vi "NBFM Modulation Demo (Single Tone) - Basic.vi"() -> ()   [LabVIEW 2013]
uses:
  <vilib>/addons/Modulation/Analog/MT Passband PLL.vi
  <vilib>/express/express analysis/Spectral/Block/exnSpectralBlock spectral measurements power poly.vi
  <vilib>/express/express analysis/Spectral/Block/exnSpectralBlock spectral measurements power DDT.vi
  <vilib>/express/express analysis/Spectral/XNode/ExpressSpectralMeasurementsBlockNode.xnode
  <vilib>/addons/Modulation/niAMT.lvlib
panel:
  out "estimated carrier frequency (Hz)":dbl
  in  "Mod. Freq.":dbl=2000.0 caption="Frequency"
  in  "WAV SR":dbl=44100.0 caption="dt"
  in  "LPF Cut-Off":dbl=10000.0 caption="Lower Cut-Off"
  in  "AWGN (dB)":dbl(slide)=30.0 caption="Standard deviation" scale=-20.0..50.0
  out "Recovered Signal":dynamicdata(graph)
  out "Baseband":dynamicdata(graph)
  out "FM FFT":dynamicdata(graph)
  out "FM Wave":dynamicdata(graph)
  in  "Carrier Amp.":dbl=1.0 caption="Amplitude"
  in  "stop":bool
  in  "Frequency Deviation":dbl(slide)=400.0 scale=0.0..400.0
  in  "Carrier Freq.":dbl=100000.0 caption="Frequency"
  # "Frequency Modulation"
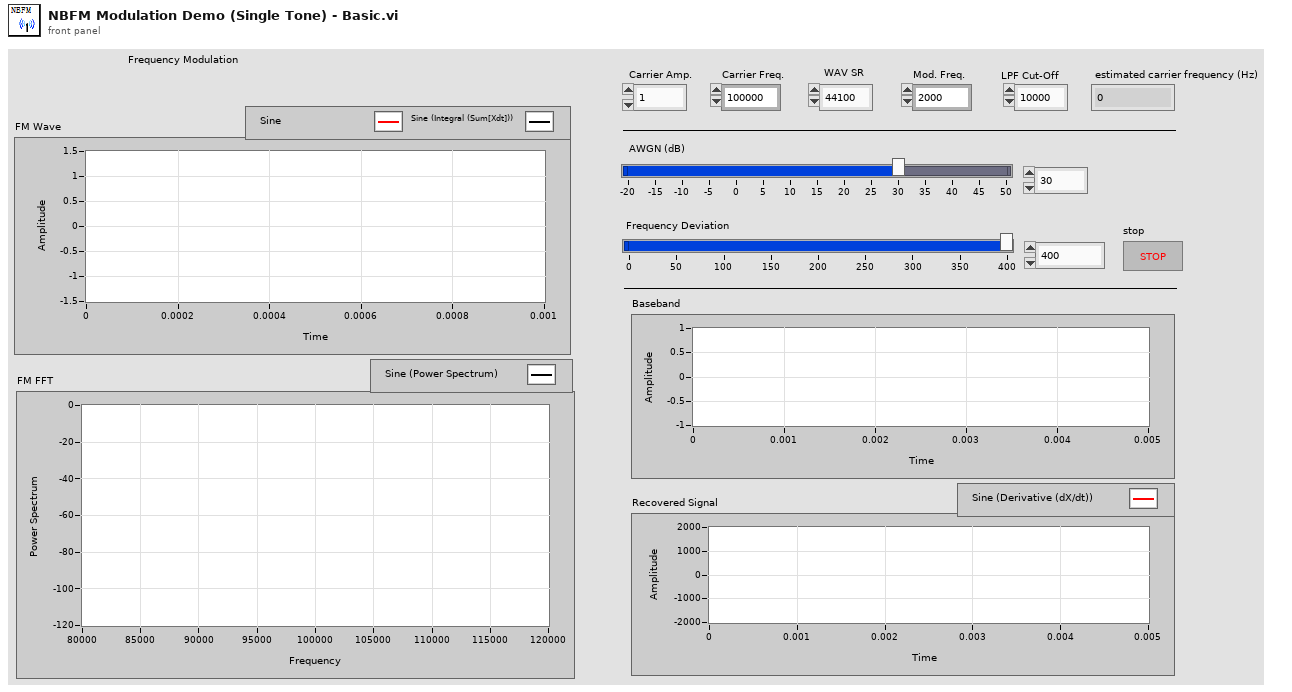
[diagram p1: front panel]
types:
  T1 = cluster{"averaging mode":u16, "weighting mode":u16, "number of averages":u32}
  T2 = cluster{"dB On (F)":bool, "unwrap phase (F)":bool, "convert to degree (F)":bool}
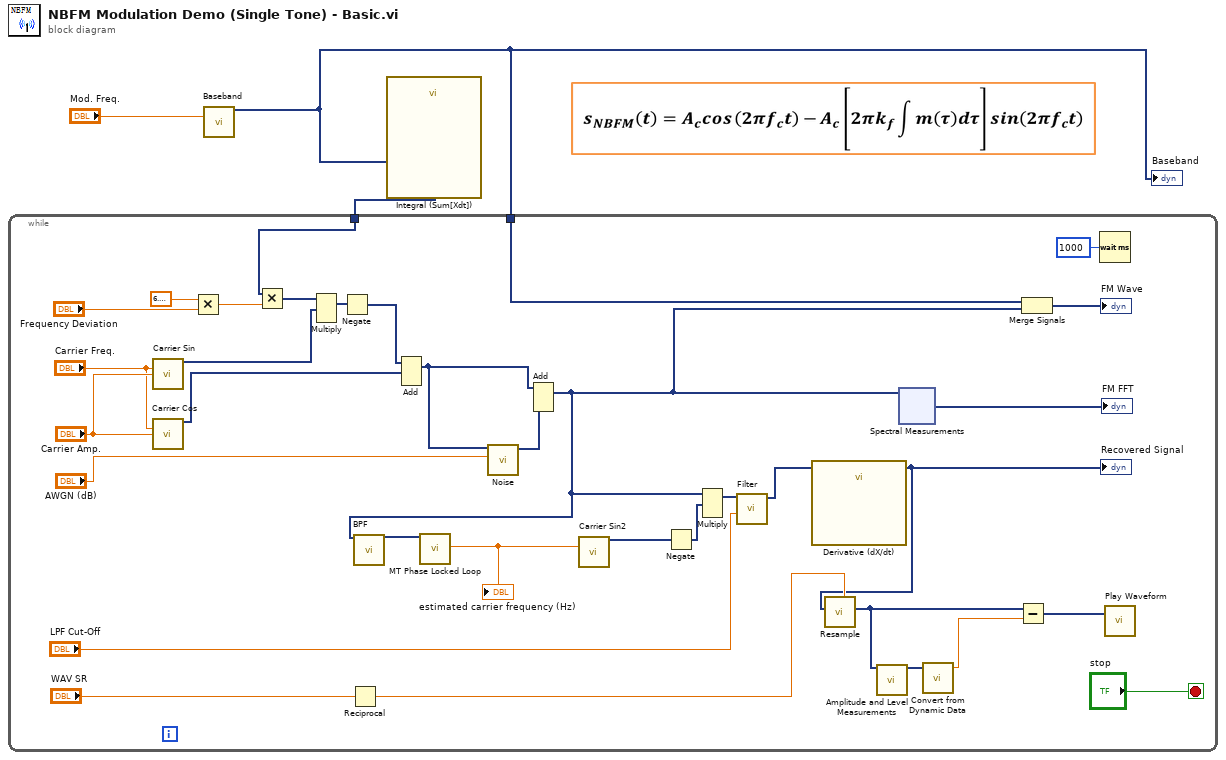
[diagram p0: block diagram]
diagram:
  n1 = call "Baseband"("Frequency"="Mod. Freq.") -> ("Sine"=w1:dynamicdata)  [unwired: 13 in, 1 out]
  "Baseband" <- w1
  n2 = call "Integral (Sum[Xdt])"("Signals"=w1) -> ("Result"=w2:dynamicdata)  [unwired: 5 in, 1 out]
  n3 = while {
    tunnel: w2 -> [w30]
    tunnel: w1 -> [w34]
    stop <- "stop" stop-if-true
    n4 = call "Carrier Sin"("Frequency"="Carrier Freq.", "Amplitude"="Carrier Amp.") -> ("Sine"=w28:dynamicdata)  [unwired: 12 in, 1 out]
    n5 = call "Carrier Cos"("Frequency"="Carrier Freq.", "Amplitude"="Carrier Amp.") -> ("Sine"=w23:dynamicdata)  [unwired: 12 in, 1 out]
    n6 = Multiply(x=6.283185307179586, y="Frequency Deviation") -> (x*y=w31:dbl)
    n7 = Multiply(x=w30, y=w31) -> (x*y=w29:dynamicdata)
    n8 = Multiply(1:w28, 2:w29) -> (0:w25:dynamicdata)  [unwired: 1 in, 1 out]
    n9 = Negate(x=w25) -> (-x=w24:dynamicdata)
    n10 = Reciprocal(x="WAV SR") -> (1/x=w10:dbl)
    n11 = Add(1:w23, 2:w24) -> (0:w20:dynamicdata)  [unwired: 1 in, 1 out]
    n12 = call "Noise.vi"("AWGN (dB)"="AWGN (dB)", "Dynamic Data"=w20) -> ("DC with Gaussian Noise"=w21:dynamicdata)  [unwired: 9 in]
    n13 = Add(1:w21, 2:w20) -> (0:w5:dynamicdata)  [unwired: 1 in, 1 out]
    n14 = call "BPF"("Signal"=w5) -> ("Filtered Signal"=w18:dynamicdata)  [unwired: 9 in, 1 out]
    n15 = call-poly <vilib>:"MT Phase Locked Loop.vi"("passband waveform"=w18) -> ("estimated carrier frequency (Hz)"=w4:dbl)  [unwired: 10 in, 4 out]
    "estimated carrier frequency (Hz)" <- w4
    n16 = call "Carrier Sin2"("Frequency"=w4) -> ("Sine"=w17:dynamicdata)  [unwired: 13 in, 1 out]
    n17 = Negate(x=w17) -> (-x=w16:dynamicdata)
    n18 = Multiply(1:w16, 2:w5) -> (0:w14:dynamicdata)  [unwired: 1 in, 1 out]
    n19 = call "Filter"("Lower Cut-Off"="LPF Cut-Off", "Signal"=w14) -> ("Filtered Signal"=w13:dynamicdata)  [unwired: 8 in, 1 out]
    n20 = call "Derivative (dX/dt)"("Signals"=w13) -> ("Result"=w9:dynamicdata)  [unwired: 5 in, 1 out]
    "Recovered Signal" <- w9
    n21 = call "Resample"("dt"=w10, "Signals"=w9) -> ("Resampled Signals"=w8:dynamicdata)  [unwired: 7 in, 2 out]
    n22 = call "Amplitude and Level Measurements"("Signals"=w8) -> ("Mean (DC)"=w11:dynamicdata)  [unwired: 13 in, 1 out]
    n23 = xnode "Spectral Measurements"("Signals"=w5) -> ("Power Spectrum"=→"FM FFT":dynamicdata)  [unwired: 1 in, 1 out]
    n24 = call "Convert from Dynamic Data"("Dynamic Data Type"=w11) -> ("Scalar"=w7:dbl)  [unwired: 3 in]
    n25 = Subtract(x=w8, y=w7) -> (x-y=w6:dynamicdata)
    n26 = Merge Signals(w34, w5) -> (→"FM Wave":dynamicdata)
    n27 = Wait (ms)(milliseconds to wait=u32 1000) -> ()  [unwired: 1 out]
    n28 = call "Play Waveform"("Data"=w6) -> ()  [unwired: 18 in, 1 out]
  }
